vi "Parse Data.vi"(8 "error in":errorcluster, 11 "Data In":string) -> (0 "error out":errorcluster, 2 "Result?":bool, 3 "Result Data Out":string)   [LabVIEW 2017]
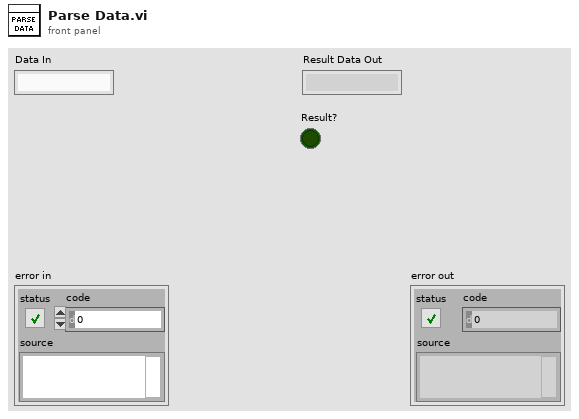
[diagram p1: front panel]
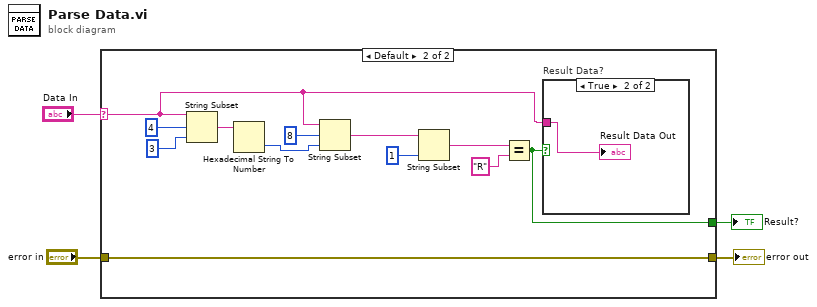
[diagram p0: block diagram]
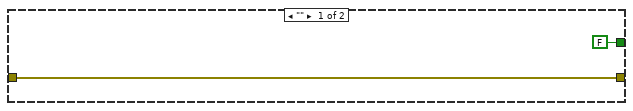
[diagram p2: hidden frame]
diagram:
  n1 = case shown="Default" "Data In" {
    selector: "Data In" -> [_ w7]
    tunnel: [w6 w9] -> w3
    tunnel: "error in" -> [w6 w9]
    tunnel: [FALSE w8] -> w1
    frame "" {
    }
    frame Default {
      n2 = String Subset(string=w7, offset (0)=4, length (rest)=3 ("length (rest)")) -> (substring=w15:string)
      n3 = Hexadecimal String To Number(string=w15) -> (number=w11:u32)  [unwired: 2 in, 1 out]
      n4 = String Subset(string=w7, offset (0)=8, length (rest)=w11) -> (substring=w18:string)
      n5 = String Subset(string=w18, length (rest)=1 ("length (rest)")) -> (substring=w10:string)  [unwired: 1 in]
      n6 = Equal?(x=w10, y="R") -> (x = y?=w8:bool)
      n7 = case "Result Data?" shown="True" w8 {
        tunnel: w7 -> [_ w19]
        frame False {
        }
        frame True {
          "Result Data Out" <- w19
        }
      }
    }
  }
  "error out" <- w3
  "Result?" <- w1
